vi "DSF.Transceiver.UDP.Get Transfer Group Names.vi"(11 "UDP Transceiver in":refnum<class "DSF.Transceiver.UDP.lvclass">) -> (2 "Transfer Group names":string[](array[string]), 3 "UDP Transceiver out":refnum<class "DSF.Transceiver.UDP.lvclass">)   [LabVIEW 2017, in "DSF.Transceiver.UDP.lvlib" / "DSF.Transceiver.UDP.lvclass"]
uses:
  DSF.Transceiver.UDP.lvclass
  DSF.Transceiver.UDP.lvclass/DSF.Transceiver.UDP.ctl
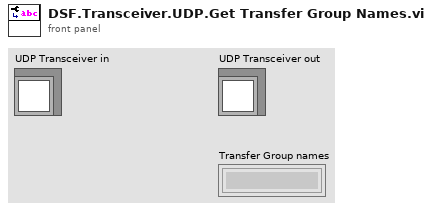
[diagram p1: front panel]
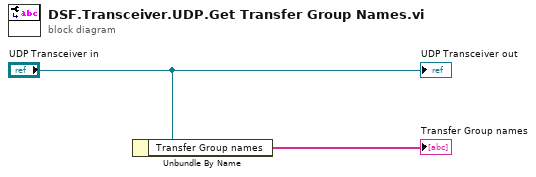
[diagram p0: block diagram]
diagram:
  n1 = Unbundle By Name("UDP Transceiver in") -> ("Transfer Group names"=→"Transfer Group names":string[])
  "UDP Transceiver out" <- "UDP Transceiver in"
